vi "Get Magnitude and Phase Header - SParam_VST.vi"(9 "Magnitude Units":i32(ring) items=["dB", "Linear"], 10 "x-axis":string, 11 "Plot Names":string[](array[string])) -> (3 "Header":string[](array[string]))   [LabVIEW 2023, in "FPT_SParam_VST UI.lvlib"]
uses:
  FPT_SParam_VST UI.lvlib
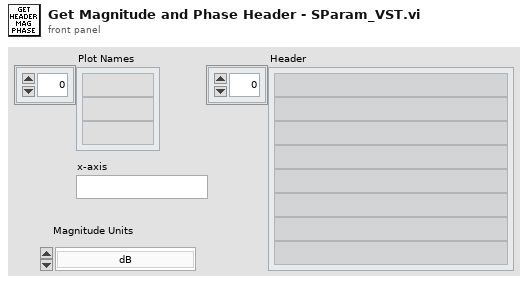
[diagram p1: front panel]
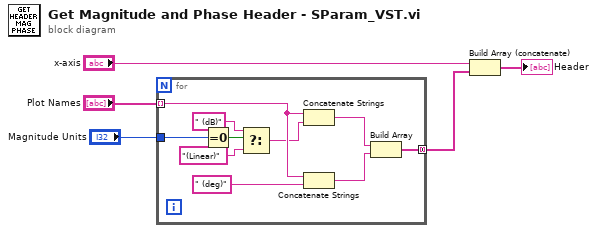
[diagram p0: block diagram]
diagram:
  n1 = for {
    tunnel: "Plot Names" -> [w15] mode=indexing
    tunnel: [w12] -> w2 mode=concatenating
    tunnel: "Magnitude Units" -> [w9]
    n2 = Equal To 0?(x=w9) -> (x = 0?=w8:bool)
    n3 = Select(t=" (dB)" ("string"), s=w8, f="(Linear)") -> (s? t:f=w11:string)
    n4 = Concatenate Strings(w15, w11) -> (w6:string)
    n5 = Concatenate Strings(w15, " (deg)" ("string")) -> (w13:string)
    n6 = Build Array(w6, w13) -> (w12:string[])
  }
  n7 = Build Array (concatenate)("x-axis", w2) -> (→"Header":string[])
